vi "GetStartRowCol.vi"(11 "Cell Type Data":string[][](array[string])) -> (2 "#Cols Empty":i32, 3 "#Rows Empty":i32)   [LabVIEW 2014]
panel:
  # "Output"
  # "Input"
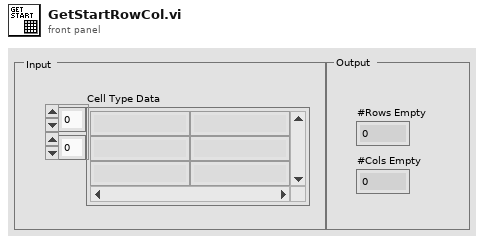
[diagram p1: front panel]
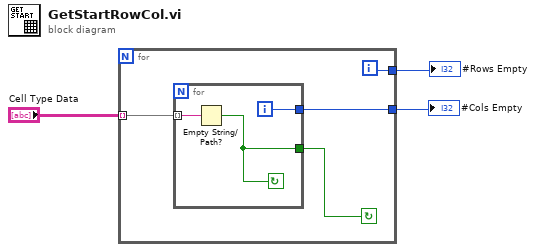
[diagram p0: block diagram]
diagram:
  n1 = for {
    tunnel: "Cell Type Data" -> [w7] mode=indexing
    tunnel: [w4] -> w3
    tunnel: [w5] -> w2
    i -> [w4]
    stop <- w6 continue-if-true
    n2 = for {
      tunnel: w7 -> [w10] mode=indexing
      tunnel: [w9] -> w6
      tunnel: [w8] -> w5
      i -> [w8]
      stop <- w9 continue-if-true
      n3 = Empty String/Path?(string/path=w10) -> (empty?=w9:bool)
    }
  }
  "#Rows Empty" <- w3
  "#Cols Empty" <- w2
